vi "Calculate Jogwheel Value.vi"(11 "Playback Position":i32) -> (2 "Jogwheel Label Image":i32, 3 "Jogwheel Position":i32)   [LabVIEW 2019, in "User Interface.lvlib"]
doc: "Calculate the jogwheel value and label value based on the current playback position."
uses:
  User Interface.lvlib
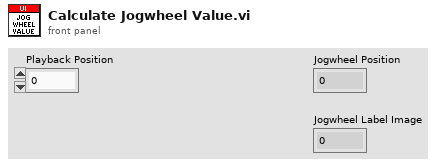
[diagram p1: front panel]
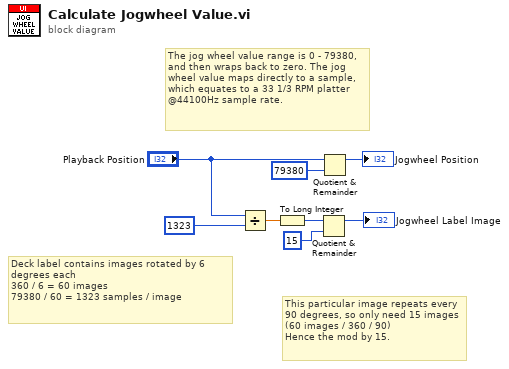
[diagram p0: block diagram]
diagram:
  # "This particular image repeats every 90 degrees, so only need 15 images (60 images / 360 / 90)\nHence the mod by 15."
  # "Deck label contains images rotated by 6 degrees each\n360 / 6 = 60 images\n79380 / 60 = 1323 samples / image"
  # "The jog wheel value range is 0 - 79380, and then wraps back to zero. The jog wheel value maps directly to a sample, which equates to a 33 1/3 RPM platter @44100Hz sample rate."
  n1 = Divide(x="Playback Position", y=1323) -> (x/y=w7:dbl)
  n2 = To Long Integer(number=w7) -> (32bit integer=w5:i32)
  n3 = Quotient & Remainder(x=w5, y=15) -> (x-y*floor(x/y)=→"Jogwheel Label Image":i32)  [unwired: 1 out]
  n4 = Quotient & Remainder(x="Playback Position", y=79380) -> (x-y*floor(x/y)=→"Jogwheel Position":i32)  [unwired: 1 out]
